vi "Subscription Policy Initialize.vi"(8 "error in (no error)":errorcluster, 9 "Last Publish Time":timestamp, 10 "Last Topic Value":variant, 11 "ValueChangeSubscription In":refnum<class "ValueChangeSubscription.lvclass">) -> (0 "error out":errorcluster, 3 "ValueChangeSubscription Out":refnum<class "ValueChangeSubscription.lvclass">)   [LabVIEW 2015, in "Mediator.lvlib" / "ValueChangeSubscription.lvclass"]
uses:
  ValueChangeSubscription.lvclass
  ValueChangeSubscription.lvclass/ValueChangeSubscription.ctl
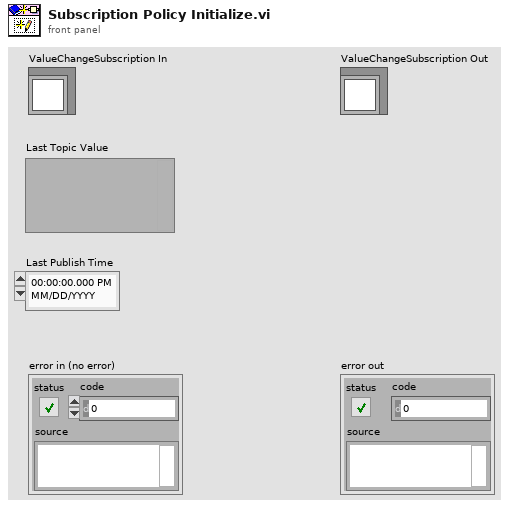
[diagram p1: front panel]
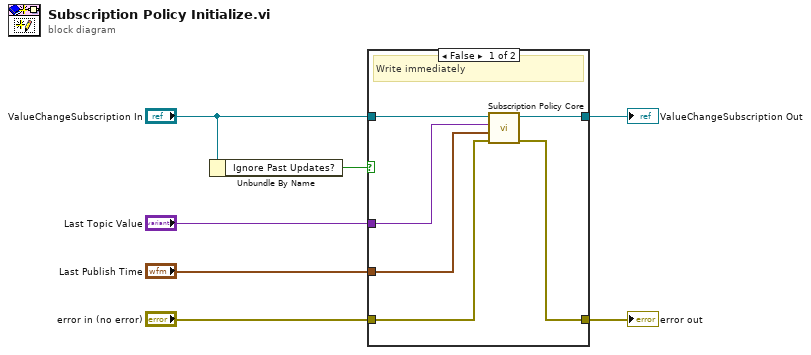
[diagram p0: block diagram]
diagram:
  n1 = Unbundle By Name("ValueChangeSubscription In") -> ("Ignore Past Updates?"=w5:bool)
  n2 = case shown="False" w5 {
    tunnel: "ValueChangeSubscription In" -> [w13 w15]
    tunnel: [w12 w15] -> w6
    tunnel: "Last Topic Value" -> [w9 _]
    tunnel: "Last Publish Time" -> [w10 _]
    tunnel: "error in (no error)" -> [w11 w14]
    tunnel: [w8 w14] -> w1
    frame False {
      # "Write immediately"
      n3 = call-dynamic "Subscription Policy Core.vi"("error in (no error)"=w11, "Publish Time"=w10, "New Topic Value"=w9, "ValueChangeSubscription In"=w13) -> ("error out"=w8:errorcluster, "ValueChangeSubscription Out"=w12:refnum<class "ValueChangeSubscription.lvclass">)  [unwired: 6 in]
    }
    frame True {
      # "Ignore past updates"
    }
  }
  "error out" <- w1
  "ValueChangeSubscription Out" <- w6
